vi "sum_gist11.vi"(1 "hist2":cluster{i16[], i32[]}, 2 "hist1":cluster{i16[], i32[]}) -> (0 "hist1+2":cluster{i16[], i32[]})   [LabVIEW 2010]
panel:
  # "Сложение двух гистограмм"
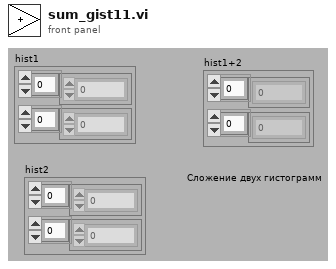
[diagram p1: front panel]
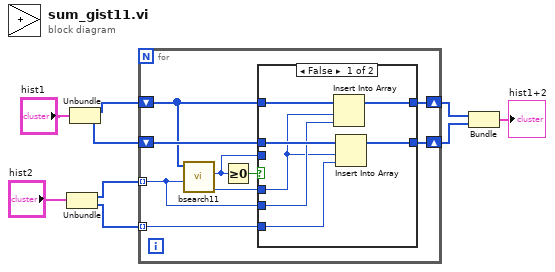
[diagram p0: block diagram]
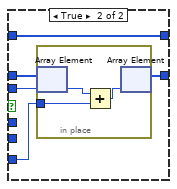
[diagram p2: hidden frame]
diagram:
  n1 = Unbundle("hist2") -> (w7:i16[], w6:i32[])
  n2 = Unbundle("hist1") -> (w5:i16[], w4:i32[])
  n3 = for {
    tunnel: w7 -> [w11] mode=indexing
    tunnel: w6 -> [w16] mode=indexing
    shift-right: [w13] -> w3
    shift-left: w5 -> [w12]
    shift-right: [w14] -> w2
    shift-left: w4 -> [w17]
    n4 = call "bsearch11.vi"("val"=w11, "Array"=w12) -> ("a"=w10:i32, "idx"=w15:i32)  [unwired: 4 in]
    n5 = Greater Or Equal To 0?(x=w15) -> (x >= 0?=w18:bool)
    n6 = case shown="False" w18 {
      tunnel: w17 -> [w23 w30]
      tunnel: w16 -> [w20 w29]
      tunnel: w15 -> [_ w28]
      tunnel: [w22 w27] -> w14
      tunnel: [w24 w26] -> w13
      tunnel: w12 -> [w25 w26]
      tunnel: w11 -> [w21 _]
      tunnel: w10 -> [w19 _]
      frame False {
        n7 = Insert Into Array(array=w25, index=w19, new element=w21) -> (w24:i16[])
        n8 = Insert Into Array(array=w23, index=w19, new element=w20) -> (w22:i32[])
      }
      frame True {
        n9 = in-place {
          in-place-border: w29 -> [w31]
          n10 = in-place-array #1(w30, w28) -> (w33:i32)
          n11 = Add(x=w33, y=w31) -> (x+y=w32:i32)
          n12 = in-place-array #1(w32) -> (w27:i32[])  [unwired: 1 out]
        }
      }
    }
  }
  n13 = Bundle(w3, w2) -> (→"hist1+2":cluster{i16[], i32[]})  [unwired: 1 in]
